vi "Create Dynamic VI In Class.vi"(8 "error in (no error)":errorcluster, 9 "New VI Path":path, 10 "LVClassLibrary in":refnum<vi>, 11 "RPC Method Name":string) -> (0 "error out":errorcluster, 3 "dynamic member vi out":refnum<vi>)   [LabVIEW 2019, in "gRPC Template Creation Utility.lvlib"]
uses:
  gRPC Template Creation Utility.lvlib
panel:
  out "LVClassLibrary out":refnum<vi>
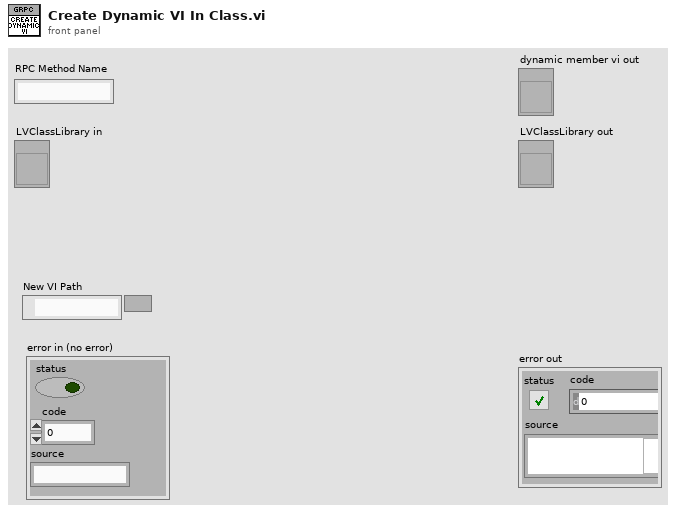
[diagram p1: front panel]
types:
  T1 = enum16{"Invalid Wire Rule", "Required", "Recommended", "Optional", "Dynamic Dispatch"}
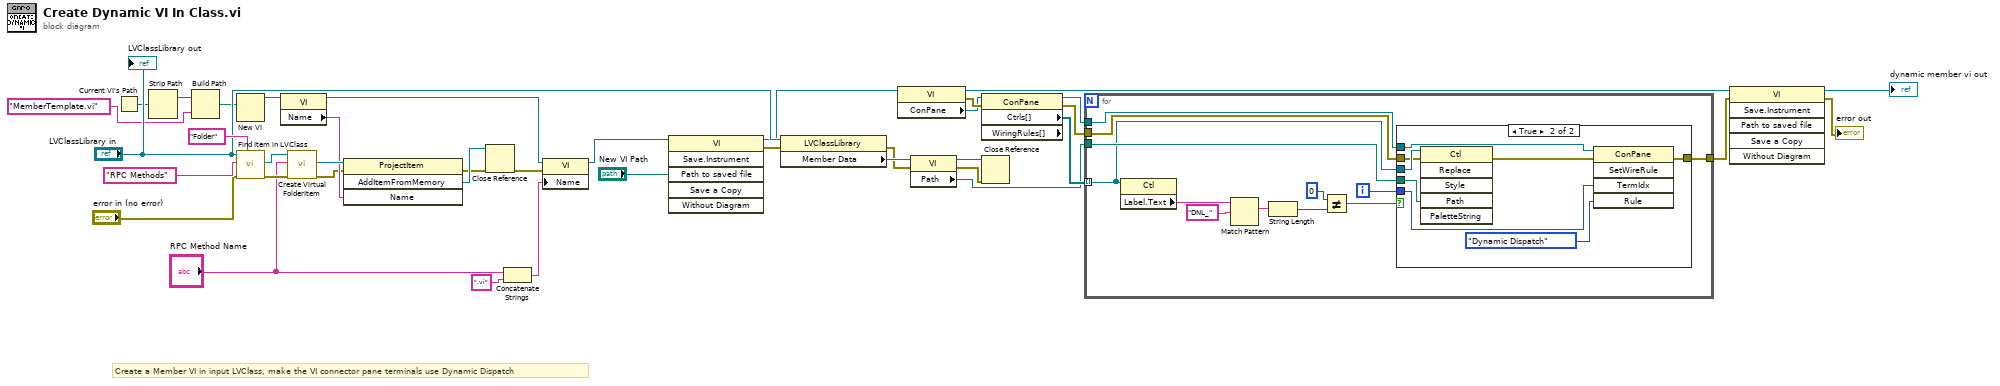
[diagram p0: block diagram]
diagram:
  # "Create a Member VI in input LVClass, make the VI connector pane terminals use Dynamic Dispatch"
  n1 = Current VI's Path() -> (path=w8:path)
  n2 = Strip Path(path=w8) -> (stripped path=w6:path)  [unwired: 1 out]
  n3 = Build Path(base path=w6, name or relative path="MemberTemplate.vi") -> (appended path=w5:path)
  n4 = New VI(10:w5) -> (3:w26:refnum<vi>)  [unwired: 6 in, 1 out]
  n5 = call "Find Item in LVClass.vi"("Item Type"="Folder", "error in (no error)"="error in (no error)", "Item Name"="RPC Methods", "Class Item in"="LVClassLibrary in") -> ("error out"=w21:errorcluster, "Project Item (Class Item)"=w28:refnum<vi>)  [unwired: 4 in, 2 out]
  n6 = property class="VI"(reference=w26) -> (reference out=w15:refnum<vi>, "Name"=w25:string)  [unwired: 1 in, 1 out]
  n7 = call "Create Virtual FolderItem.vi"("error in (no error)"=w21, "Folder Name"="RPC Method Name", "ProjectItem in"=w28) -> ("error out"=w20:errorcluster, "FolderItem reference out"=w27:refnum<vi>)  [unwired: 5 in, 2 out]
  n8 = invoke class="ProjectItem" method="AddItemFromMemory"(reference=w27, error in=w20, "Name"=w25) -> (error out=w23:errorcluster, "AddItemFromMemory"=w24:refnum<vi>)  [unwired: 1 in, 2 out]
  n9 = Close Reference(reference=w24, error in (no error)=w23) -> (error out=w19:errorcluster)
  n10 = Concatenate Strings("RPC Method Name", ".vi" ("string")) -> (w16:string)
  n11 = property class="VI"(reference=w15, error in=w19, "Name"=w16) -> (reference out=w14:refnum<vi>)  [unwired: 1 out]
  n12 = invoke class="VI" method="Save.Instrument"(reference=w14, "Path to saved file"="New VI Path") -> (reference out=w11:refnum<vi>, error out=w12:errorcluster)  [unwired: 4 in, 4 out]
  n13 = property class="LVClassLibrary"(reference="LVClassLibrary in", error in=w12) -> (error out=w2:errorcluster, "Member Data"=w38:refnum<vi>)  [unwired: 1 out]
  n14 = property class="VI"(reference=w11) -> (reference out=w32:refnum<vi>, error out=w39:errorcluster, "ConPane"=w37:refnum<vi>)  [unwired: 1 in]
  n15 = property class="VI"(reference=w38, error in=w2) -> (reference out=w3:refnum<vi>, error out=w1:errorcluster, "Path"=w34:path)
  n16 = property class="ConPane" props=["Ctrls[]", "WiringRules[]"](reference=w37, error in=w39) -> (reference out=w33:refnum<vi>, error out=w4:errorcluster, "Ctrls[]"=w35:refnum<vi>[])  [unwired: 1 out]
  n17 = Close Reference(reference=w3, error in (no error)=w1) -> ()  [unwired: 1 out]
  n18 = for {
    tunnel: w35 -> [w47] mode=indexing
    tunnel: w34 -> [w51]
    tunnel: w33 -> [w50]
    tunnel: [w48] -> w31
    tunnel: w4 -> [w40]
    i -> [w49]
    n19 = property class="Ctl"(reference=w47) -> ("Label.Text"=w46:string)  [unwired: 1 in, 2 out]
    n20 = Match Pattern(string=w46, regular expression="DNL_") -> (match substring=w44:string)  [unwired: 1 in, 3 out]
    n21 = String Length(string=w44) -> (length=w43:i32)
    n22 = Not Equal?(x=0, y=w43) -> (x != y?=w41:bool)
    n23 = case shown="True" w41 {
      tunnel: w47 -> [_ w60]
      tunnel: w51 -> [_ w59]
      tunnel: w50 -> [_ w58]
      tunnel: w49 -> [_ w56]
      tunnel: [w52 w54] -> w48
      tunnel: w40 -> [w52 w53]
      frame False {
      }
      frame True {
        n24 = invoke class="Ctl" method="Replace"(reference=w60, error in=w53, "Path"=w59) -> (error out=w55:errorcluster)  [unwired: 3 in, 5 out]
        n25 = invoke class="ConPane" method="SetWireRule"(reference=w58, error in=w55, "TermIdx"=w56, "Rule"=T1."Dynamic Dispatch") -> (error out=w54:errorcluster)  [unwired: 1 in, 4 out]
      }
    }
  }
  n26 = invoke class="VI" method="Save.Instrument"(reference=w32, error in=w31) -> (reference out=→"dynamic member vi out":refnum<vi>, error out=→"error out":errorcluster)  [unwired: 4 in, 4 out]
  "LVClassLibrary out" <- "LVClassLibrary in"
